vi "configure image source.vi"(8 "error in (no error)":errorcluster) -> (0 "error out":errorcluster, 3 "image source parameters":T3={"Aquisition Type"=enum."IMAQ", "Interface Name"="img0", "use roi"=FALSE, "ROI"={"left"=0, "top"=0, "width"=0, "height"=0}, "camera name"="", "AVI Path"=path "", "mmf path"=path "", "stub"="", "Field Width (0 disables 0 padding)"=0, "extension"="jpg", "inter-frame interval (ms)"=200.0})   [LabVIEW 2021]
uses:
  <vilib>/userDefined/High Color/IMAQdx.ctl
panel:
  in  "path to image from stack":path
  in  "inter-frame interval (ms)":dbl=200.0
  in  "extension":string="jpg"
  in  "Field Width (0 disables 0 padding)":u8
  in  "stub":string
  in  "mmf path":path
  in  "AVI Path":path
  in  "camera name":T1="cam0"
  in  "ROI":T2
  in  "use roi":bool
  in  "Interface Name":string="img0"
  in  "done":bool
  in  "Aquisition Type":enum16{"IMAQ", "IMAQdx", "AVI", "MMF", "STACK"}(ring)
  # "For IMAQ or IMAQdx, configure camera using NI Measurement and Automation Explorer"
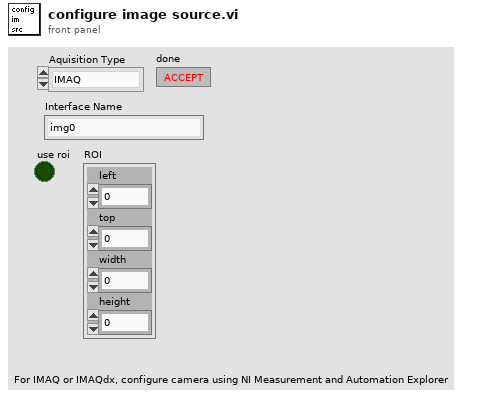
[diagram p1: front panel]
types:
  T1 = typedef "IMAQdx.ctl" = refnum<k21>
  T2 = cluster{"left":u16, "top":u16, "width":u16, "height":u16}
  T3 = cluster{"Aquisition Type":enum16{"IMAQ", "IMAQdx", "AVI", "MMF", "STACK"}, "Interface Name":string, "use roi":bool, "ROI":cluster{"left":u16, "top":u16, "width":u16, "height":u16}, "camera name":T1, "AVI Path":path, "mmf path":path, "stub":string, "Field Width (0 disables 0 padding)":u8, "extension":string, "inter-frame interval (ms)":dbl}
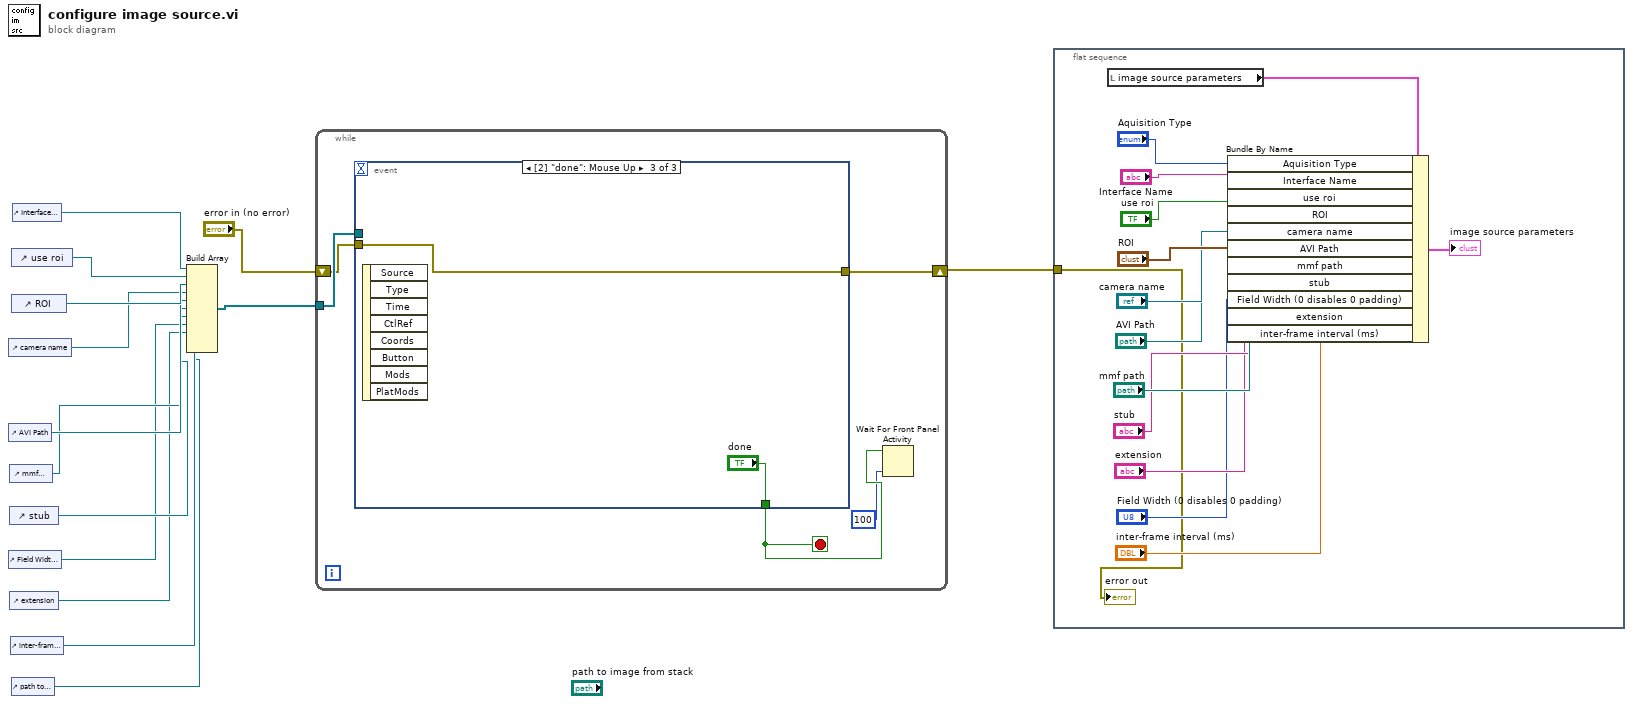
[diagram p0: block diagram]
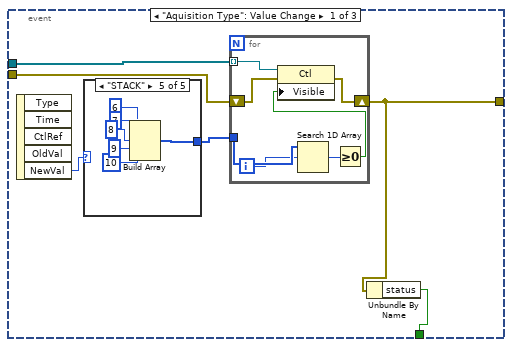
[diagram p2: hidden frame]
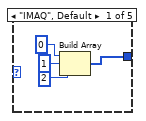
[diagram p3: hidden frame]
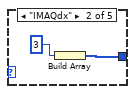
[diagram p4: hidden frame]
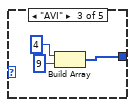
[diagram p5: hidden frame]
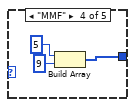
[diagram p6: hidden frame]
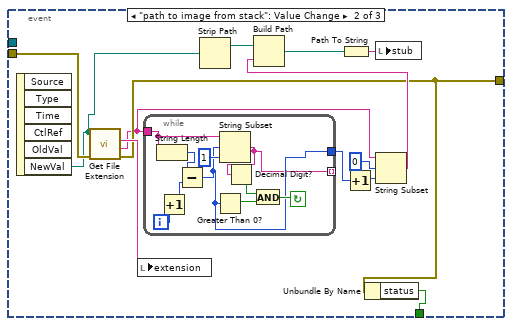
[diagram p7: hidden frame]
diagram:
  n1 = control-ref of="camera name"() -> (w12:refnum<vi>)
  n2 = control-ref of="AVI Path"() -> (w11:refnum<vi>)
  n3 = control-ref of="Field Width (0 disables 0 padding)"() -> (w8:refnum<vi>)
  n4 = control-ref of="mmf path"() -> (w10:refnum<vi>)
  n5 = control-ref of="stub"() -> (w9:refnum<vi>)
  n6 = control-ref of="extension"() -> (w7:refnum<vi>)
  n7 = control-ref of="inter-frame interval (ms)"() -> (w6:refnum<vi>)
  n8 = control-ref of="use roi"() -> (w14:refnum<vi>)
  n9 = control-ref of="ROI"() -> (w13:refnum<vi>)
  n10 = control-ref of="path to image from stack"() -> (w1:refnum<vi>)
  n11 = control-ref of="Interface Name"() -> (w4:refnum<vi>)
  n12 = Build Array(w4, w14, w13, w12, w11, w10, w9, w8, w7, w6, w1) -> (w5:refnum<vi>[])
  n13 = while {
    tunnel: w5 -> [w19]
    shift-right: [w18] -> w2
    shift-left: "error in (no error)" -> [w17]
    stop <- w16 stop-if-true
    n14 = event shown="[2] \"done\": Mouse Up" {
      selector: _ -> [_ _ _]
      dyn-events: _ -> [_ _ _]
      timeout: _ -> [_ _ _]
      tunnel: w19 -> [w24 _ _]
      tunnel: [w21 w52 w74] -> w18
      tunnel: w17 -> [w22 w61 w74]
      tunnel: [w20 w53 "done"] -> w16
      event "Aquisition Type": Value Change {
        n15 = event-data() -> ("NewVal"=w25:enum16{"IMAQ", "IMAQdx", "AVI", "MMF", "STACK"})  [unwired: 1 in, 4 out]
        n16 = case shown="\"STACK\"" w25 {
          tunnel: [w33 w37 w40 w43 w49] -> w23
          frame "IMAQ", Default {
            n17 = Build Array(0, 1 ("element"), 2 ("element")) -> (w33:i32[])
          }
          frame "IMAQdx" {
            n18 = Build Array(3) -> (w37:i32[])
          }
          frame "AVI" {
            n19 = Build Array(4, 9 ("element")) -> (w40:i32[])
          }
          frame "MMF" {
            n20 = Build Array(5, 9 ("element")) -> (w43:i32[])
          }
          frame "STACK" {
            n21 = Build Array(7 ("element"), 6 ("element"), 8, 9 ("element"), 10 ("element")) -> (w49:i32[])
          }
        }
        n22 = for {
          tunnel: w24 -> [w32] mode=indexing
          shift-right: [w31] -> w21
          shift-left: w22 -> [w30]
          tunnel: w23 -> [w29]
          i -> [w28]
          n23 = Search 1D Array(1D array=w29, element=w28) -> (index of element=w27:i32)  [unwired: 1 in]
          n24 = Greater Or Equal To 0?(x=w27) -> (x >= 0?=w26:bool)
          n25 = property class="Ctl"(reference=w32, error in=w30, "Visible"=w26) -> (error out=w31:errorcluster)  [unwired: 1 out]
        }
        n26 = Unbundle By Name(w21) -> ("status"=w20:bool)
      }
      event "path to image from stack": Value Change {
        n27 = event-data() -> ("NewVal"=w59:path)  [unwired: 1 in, 5 out]
        n28 = call <vilib>:"Get File Extension.vi"("error in (no error)"=w61, "file"=w59) -> ("error out"=w52:errorcluster, "filename without extension"=w51:string, "lowercase file extension"=w54:string)  [unwired: 5 in, 2 out]
        n29 = local write "extension"(w54) -> ()
        n30 = while {
          tunnel: w51 -> [w73]
          tunnel: [w66] -> w60
          tunnel: [w65] -> _ mode=indexing
          i -> [w71]
          stop <- w67 continue-if-true
          n31 = String Length(string=w73) -> (length=w72:i32)
          n32 = Increment(x=w71) -> (x+1=w64:i32)
          n33 = Subtract(x=w72, y=w64) -> (x-y=w66:i32)
          n34 = Greater Than 0?(x=w66) -> (x > 0?=w68:bool)
          n35 = String Subset(string=w73, offset (0)=w66, length (rest)=1 ("length (rest)")) -> (substring=w65:string)
          n36 = Decimal Digit?(1:w65) -> (0:w69:bool)
          n37 = And(x=w69, y=w68) -> (x .and. y?=w67:bool)
        }
        n38 = Strip Path(path=w59) -> (stripped path=w58:path)  [unwired: 1 out]
        n39 = Increment(x=w60) -> (x+1=w62:i32)
        n40 = Unbundle By Name(w52) -> ("status"=w53:bool)
        n41 = String Subset(string=w51, offset (0)=0, length (rest)=w62) -> (substring=w57:string)
        n42 = Build Path(base path=w58, name or relative path=w57) -> (appended path=w56:path)
        n43 = Path To String(path=w56) -> (string=w55:string)
        n44 = local write "stub"(w55) -> ()
      }
      event "done": Mouse Up {
        n45 = event-data() -> ()  [unwired: 1 in, 8 out]
      }
    }
    n46 = Wait For Front Panel Activity(1:100 ("timeout ms (-1 never timeout)"), 3:w16) -> ()  [unwired: 1 in, 1 out]
  }
  n47 = flat-sequence {
    tunnel: w2 -> [w76]
    frame #0 {
      n48 = local read "image source parameters"() -> (w89:T3)
      n49 = Bundle By Name(cluster=w89, "Aquisition Type"="Aquisition Type", "Interface Name"="Interface Name", "use roi"="use roi", "ROI"="ROI", "camera name"="camera name", "AVI Path"="AVI Path", "mmf path"="mmf path", "stub"="stub", "Field Width (0 disables 0 padding)"="Field Width (0 disables 0 padding)", "extension"="extension", "inter-frame interval (ms)"="inter-frame interval (ms)") -> (→"image source parameters":T3)
      "error out" <- w76
    }
  }
